vi "Get Wheel Parameter Names.vi"(8 "error in (no error)":errorcluster, 11 "wheel in":refnum<class "NI_Robotics_Steering Wheel.lvclass">) -> (0 "error out":errorcluster, 2 "parameter names":string[](array[string]), 3 "wheel out":refnum<class "NI_Robotics_Steering Wheel.lvclass">)   [LabVIEW 2017, in "NI_Robotics_Steering Wheel.lvclass"]
uses:
  <vilib>/robotics/Steering/Steering Wheel/NI_Robotics_Steering Wheel.lvclass
  <vilib>/robotics/Steering/Wheel/NI_Robotics_Wheel.lvclass
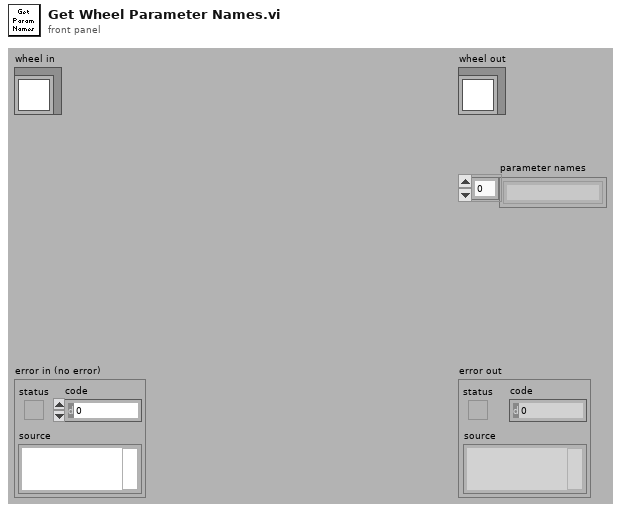
[diagram p1: front panel]
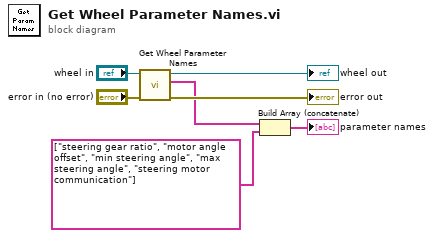
[diagram p0: block diagram]
diagram:
  n1 = call-parent "Get Wheel Parameter Names.vi"("error in (no error)"="error in (no error)", "wheel in"="wheel in") -> ("error out"=→"error out":errorcluster, "parameter names"=w2:string[], "wheel out"=→"wheel out":refnum<class "NI_Robotics_Steering Wheel.lvclass">)  [unwired: 7 in]
  n2 = Build Array (concatenate)(w2, string[] ["steering gear ratio", "motor angle offset", "min steering angle", "max steering angle", "steering motor communication"] ("parameter names")) -> (→"parameter names":string[])
